vi "Read&Write Counter.vi"(8 "error in":errorcluster, 9 "Count IN":i32, 10 "Write/Read":bool=TRUE, 11 "Path In":path=path "D:/Lens_Tuning/VVDN/LensTuningCounter") -> (0 "error out":errorcluster, 3 "Count OUT":i32)   [LabVIEW 2019]
panel:
  in  "Data Type":i32
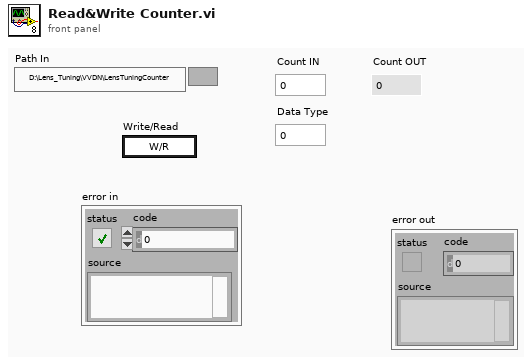
[diagram p1: front panel]
types:
  T1 = enum16{"open", "replace", "create", "open or create", "replace or create", "replace or create with confirmation"}
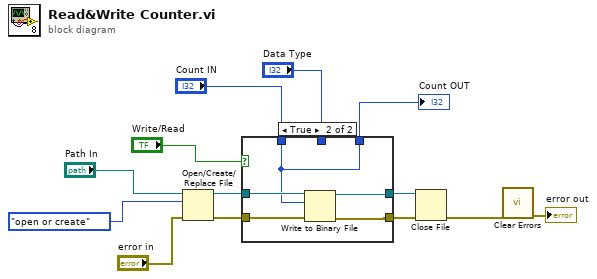
[diagram p0: block diagram]
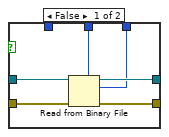
[diagram p2: hidden frame]
diagram:
  n1 = Open/Create/Replace File(file path (use dialog)="Path In", error in="error in", operation (0:open)=T1."open or create") -> (refnum out=w13:refnum<file>, error out=w11:errorcluster)  [unwired: 3 in, 1 out]
  n2 = case shown="True" "Write/Read" {
    tunnel: w13 -> [w19 w24]
    tunnel: [w18 w22] -> w12
    tunnel: w11 -> [w17 w23]
    tunnel: [w16 w21] -> w10
    tunnel: "Count IN" -> [_ w20]
    tunnel: "Data Type" -> [w15 _]
    tunnel: [w14 w20] -> w3
    frame False {
      n3 = Read from Binary File(5:w15, 8:w17, 11:w19) -> (0:w16:errorcluster, 2:w14:i32, 3:w18:refnum<file>)  [unwired: 3 in, 1 out]
    }
    frame True {
      n4 = Write to Binary File(file (use dialog)=w24, data=w20, error in=w23) -> (refnum out=w22:refnum<file>, error out=w21:errorcluster)  [unwired: 3 in, 1 out]
    }
  }
  "Count OUT" <- w3
  n5 = Close File(refnum=w12, error in=w10) -> (error out=w2:errorcluster)  [unwired: 1 out]
  n6 = call <vilib>:"Clear Errors.vi"("error in (no error)"=w2) -> ("error out"=→"error out":errorcluster)  [unwired: 5 in, 1 out]
